vi "niFpgaFFTSimModelOutsideSCTLCoreWrapper.vi"(0 "real data in":fxp<+/-,16,1>, 1 "reset":bool, 5 "imaginary data in":fxp<+/-,16,1>) -> (3 "data index":u16, 4 "real data out":fxp<+/-,32,16> format="%.21g", 6 "imaginary data out":fxp<+/-,32,16> format="%.21g", 8 "output valid":bool)   [LabVIEW 2017]
uses:
  <vilib>/rvi/Analysis/measure/FFT/simModelSupport/niFPGA FFT Outside SCTL Sim Properties.ctl
  <vilib>/rvi/Analysis/measure/FFT/simModelSupport/niFPGA FFT Sim Types.ctl
  <vilib>/rvi/Analysis/measure/FFT/simModelSupport/niFpgaFFTSimArithmeticProperties.ctl
  <vilib>/rvi/Analysis/measure/FFT/simModelSupport/niFpgaFFTSimDfxp.ctl
  <vilib>/fxp/LVFixedPointQuantizationPolicyTypeDef.ctl
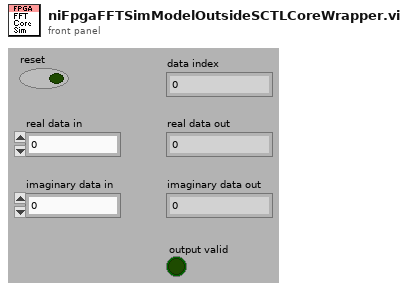
[diagram p1: front panel]
types:
  T1 = typedef "niFPGA FFT Outside SCTL Sim Properties.ctl" = cluster{"number of stages":u8, "twiddle over 16?":bool, "forward":bool, "butterfly delay":u16, "N/2":u16, "scale factor":i32, "add control logic register":bool, "switch delay":u16, "Execution Constants":cluster{"N/2-1":u16, "(N/2)*K + 1":u16, "N-1":u16, "total latency":u16, "K - 1":u8, "K - 16":i8, "K - 17":i8}, "FFT fxp types":T2}
  T2 = typedef "niFPGA FFT Sim Types.ctl" = cluster{"mult output type":T3, "internal type":T3, "twid type":T3, "sub output type":T3}
  T3 = typedef "niFpgaFFTSimArithmeticProperties.ctl" = cluster{"Output Type":T4, "Adapt To Source?":bool, "Rounding Mode":T5}
  T4 = typedef "niFpgaFFTSimDfxp.ctl" = cluster{"U64 Rep":u64, "Signed?":bool, "Word Length":i32, "Integer Word Length":i32}
  T5 = typedef "LVFixedPointQuantizationPolicyTypeDef.ctl" = enum32{"Truncate", "Round-Half-Up (Asymmetric)", "Round-Half-Even"}
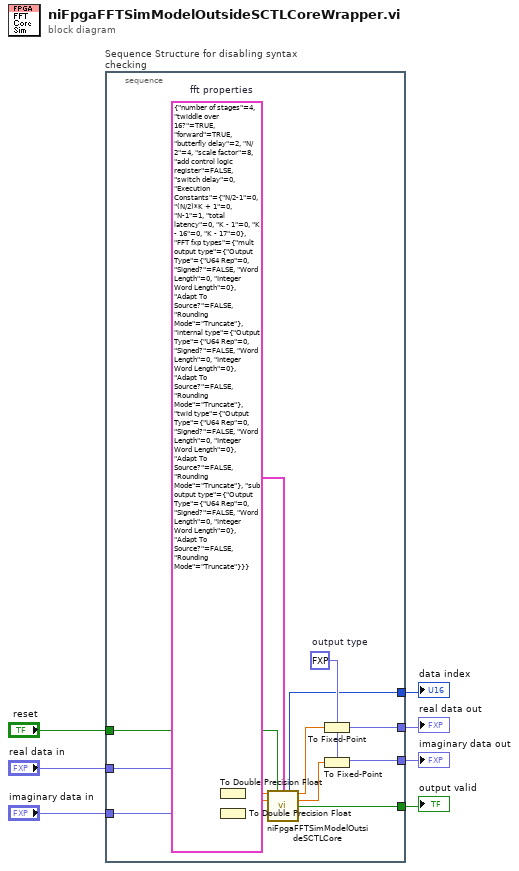
[diagram p0: block diagram]
diagram:
  n1 = stacked-sequence "Sequence Structure for disabling syntax checking" {
    tunnel: [w14] -> w7
    tunnel: [w13] -> w6
    tunnel: [w12] -> w5
    tunnel: [w11] -> w4
    tunnel: "reset" -> [w10]
    tunnel: "real data in" -> [w9]
    tunnel: "imaginary data in" -> [w8]
    frame #0 {
      w16 = T1 {"number of stages"=4, "twiddle over 16?"=TRUE, "forward"=TRUE, "butterfly delay"=2, "N/2"=4, "scale factor"=8, "add control logic register"=FALSE, "switch delay"=0, "Execution Constants"={"N/2-1"=0, "(N/2)*K + 1"=0, "N-1"=1, "total latency"=0, "K - 1"=0, "K - 16"=0, "K - 17"=0}, "FFT fxp types"={"mult output type"={"Output Type"={"U64 Rep"=0, "Signed?"=FALSE, "Word Length"=0, "Integer Word Length"=0}, "Adapt To Source?"=FALSE, "Rounding Mode"=enum."Truncate"}, "internal type"={"Output Type"={"U64 Rep"=0, "Signed?"=FALSE, "Word Length"=0, "Integer Word Length"=0}, "Adapt To Source?"=FALSE, "Rounding Mode"=enum."Truncate"}, "twid type"={"Output Type"={"U64 Rep"=0, "Signed?"=FALSE, "Word Length"=0, "Integer Word Length"=0}, "Adapt To Source?"=FALSE, "Rounding Mode"=enum."Truncate"}, "sub output type"={"Output Type"={"U64 Rep"=0, "Signed?"=FALSE, "Word Length"=0, "Integer Word Length"=0}, "Adapt To Source?"=FALSE, "Rounding Mode"=enum."Truncate"}}}  # fft properties
      w15 = fxp<+/-,32,16> 0.0  # output type
      n2 = To Double Precision Float(number=w9) -> (double precision float=w17:dbl)
      n3 = To Double Precision Float(number=w8) -> (double precision float=w18:dbl)
      n4 = call <vilib>:"niFpgaFFTSimModelOutsideSCTLCore.vi"("real data in"=w17, "reset"=w10, "fft properties"=w16, "imaginary data in"=w18) -> ("data index"=w14:u16, "real data out"=w19:dbl, "imaginary data out"=w20:dbl, "output valid"=w11:bool)  [unwired: 8 out]
      n5 = To Fixed-Point(fixed-point type=w15, number=w19) -> (fixed-point=w13:fxp<+/-,32,16>)
      n6 = To Fixed-Point(fixed-point type=w15, number=w20) -> (fixed-point=w12:fxp<+/-,32,16>)
    }
  }
  "output valid" <- w4
  "real data out" <- w6
  "imaginary data out" <- w5
  "data index" <- w7
